vi "Measure Voltage.vi"(8 "error in":errorcluster, 11 "6700 in":refnum<class "6700.lvclass">) -> (0 "error out":errorcluster, 2 "Voltage":dbl, 3 "6700 out":refnum<class "6700.lvclass">)   [LabVIEW 2018, in "6700.lvlib" / "6700.lvclass"]
uses:
  6700.lvclass
  6700.lvclass/6700.ctl
  <instrlib>/Agilent N6700 Series/Agilent N6700 Series.lvlib
  builds/Power_Supply.lvlibp/Power Supply.lvclass
  C:/Users/Ron.Dexter.LUMINARTECH/Desktop/builds/Power_Supply.lvlibp/Power Supply.lvclass
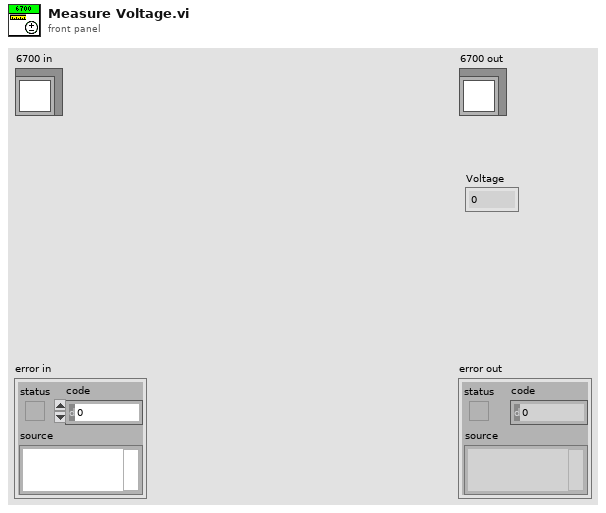
[diagram p1: front panel]
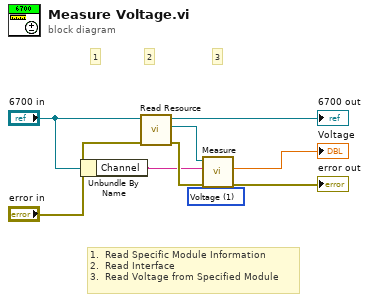
[diagram p0: block diagram]
diagram:
  w8 = 1 items=["Current", "Voltage", "Power"] ("Measurement Type (1: Voltage)")
  # "1.  Read Specific Module Information\n2.  Read Interface\n3.  Read Voltage from Specified Module"
  # "3"
  # "2"
  # "1"
  n1 = Unbundle By Name("6700 in") -> ("Channel"=w1:string)
  n2 = call "Read Resource.vi"("error in"="error in", "Power Supply in"="6700 in") -> ("error out"=w7:errorcluster, "Resource"=w6:refnum<visa-resource-name>, "Power Supply out"=→"6700 out":refnum<class "6700.lvclass">)  [unwired: 7 in]
  n3 = call <instrlib>:"Measure.vi"("error in (no error)"=w7, "Measurement Type (1: Voltage)"=w8, "Channel Name (1)"=w1, "VISA resource name"=w6) -> ("error out"=→"error out":errorcluster, "Measurement"=→"Voltage":dbl)  [unwired: 5 in, 1 out]
